vi "Safe Move.vi"(9 "Direction in":T2, 10 "Action in":T1, 11 "Map":i32[](array[numeric])) -> (1 "Direction":T2, 2 "Action":T1)   [LabVIEW 2015, in "Common.lvlib"]
uses:
  Common.lvlib
  Type Defs/Action Enum.ctl
  Type Defs/Direction Enum.ctl
  SubVIs/Read-Only Globals.vi
  Square/Square.lvclass
  Type Defs/SB Type Defs.lvlib
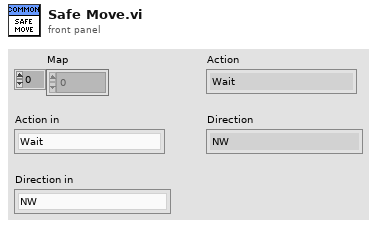
[diagram p1: front panel]
types:
  T1 = typedef "SB Type Defs.lvlib/Action Enum.ctl" = enum16{"Wait", "Move", "Attack", "Replicate"}
  T2 = typedef "SB Type Defs.lvlib/Direction Enum.ctl" = enum16{"NW", "N", "NE", "E", "SE", "S", "SW", "W"}
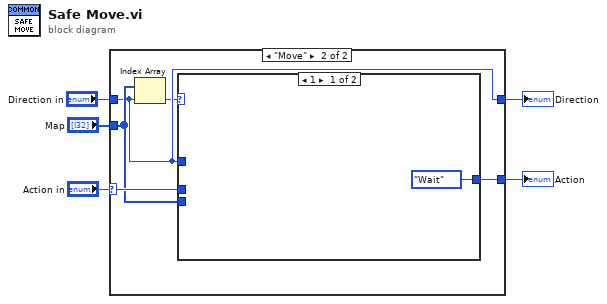
[diagram p0: block diagram]
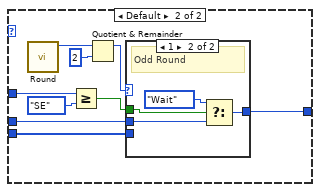
[diagram p3: hidden frame]
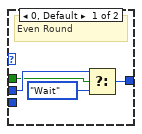
[diagram p4: hidden frame]
diagram:
  n1 = case shown="\"Move\"" "Action in" {
    selector: "Action in" -> [w7 w12]
    tunnel: "Direction in" -> [w6 w9]
    tunnel: "Map" -> [_ w10]
    tunnel: [w7 w11] -> w2
    tunnel: [w6 w9] -> w1
    frame Default {
    }
    frame "Move" {
      n2 = Index Array(array=w10, index=w9) -> (element=w8:i32)
      n3 = case shown="1" w8 {
        tunnel: w12 -> [_ w19]
        tunnel: [Action_Enum."Wait" ("Action in") w18] -> w11
        tunnel: w10 -> [_ w15]
        tunnel: w9 -> [_ w14]
        frame 1 {
        }
        frame Default {
          n4 = call "Round.vi"() -> ("Round"=w22:i32)  [unwired: 11 in]
          n5 = Greater Or Equal?(x=w14, y=Direction_Enum."SE") -> (x >= y?=w16:bool)
          n6 = Quotient & Remainder(x=w22, y=2) -> (x-y*floor(x/y)=w20:i32)  [unwired: 1 out]
          n7 = case shown="1" w20 {
            tunnel: w19 -> [w26 w30]
            tunnel: w15 -> [_ _]
            tunnel: [w25 w29] -> w18
            tunnel: w16 -> [w23 w27]
            frame 0, Default {
              # "Even Round"
              n8 = Select(t=w26, s=w23, f=Action_Enum."Wait") -> (s? t:f=w25:T1)
            }
            frame 1 {
              # "Odd Round"
              n9 = Select(t=Action_Enum."Wait" ("f"), s=w27, f=w30) -> (s? t:f=w29:T1)
            }
          }
        }
      }
    }
  }
  "Action" <- w2
  "Direction" <- w1
